vi "Example-FunctionWaveGeneration.vi"() -> ()   [LabVIEW 2018]
panel:
  in  "参数":T1={"ch"=1, "amp"=1.0, "vOffset"=0.0, "hzFrequency"=2000, "percentageSymmetry"=50.0, "degreePhase"=0.0, "func"=enum."Sine"}
  in  "output":bool=TRUE
  out "returns":i32
  out "error out":errorcluster caption="错误输出"
  in  "error in (no error)":errorcluster caption="错误输入（无错误）"
  out "ftHandle out":u64
  in  "设备索引":i32
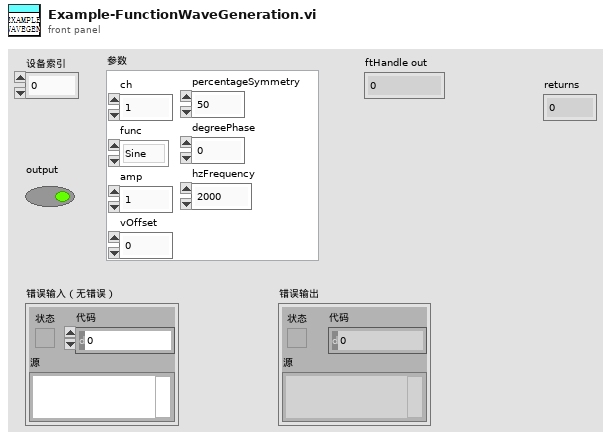
[diagram p1: front panel]
types:
  T1 = cluster{"ch":i32, "amp":dbl, "vOffset":dbl, "hzFrequency":i32, "percentageSymmetry":dbl, "degreePhase":dbl, "func":enum8{"DC", "Sine", "Square", "Triangle", "RampUp", "RampDown", "Noise", "Pulse", "Trapezium", "SinePower", "Custom", "Play"}}
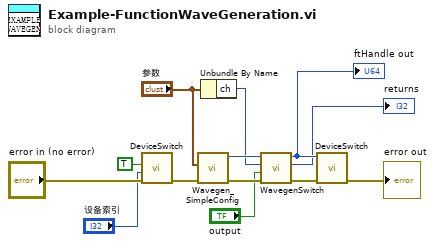
[diagram p0: block diagram]
diagram:
  n1 = call "DeviceSwitch.vi"("error in (no error)"="error in (no error)", "Device Index"="设备索引", "Open"=TRUE) -> ("error out"=w10:errorcluster)  [unwired: 4 in, 4 out]
  n2 = call "Wavegen_SimpleConfig.vi"("error in (no error)"=w10, "参数"="参数") -> ("error out"=w6:errorcluster, "ftHandle out"=w8:u64)  [unwired: 7 in, 1 out]
  n3 = Unbundle By Name("参数") -> ("ch"=w3:i32)
  n4 = call "WavegenSwitch.vi"("error in (no error)"=w6, "output"="output", "ch"=w3, "ftHandle"=w8) -> ("error out"=w7:errorcluster, "function out"=→"returns":i32, "ftHandle out"=w2:u64)  [unwired: 5 in]
  "ftHandle out" <- w2
  n5 = call "DeviceSwitch.vi"("error in (no error)"=w7, "handle"=w2) -> ("error out"=→"error out":errorcluster)  [unwired: 5 in, 4 out]
